vi "Get Slot Bus Device Function.vi"(0 "dwslot":u32, 5 "dwBus":u32, 7 "dwDevice":u32, 9 "dwFunction":u32, 11 "error in (no error)":errorcluster) -> (3 "function return":u32, 4 "dwslot out":u32, 6 "dwBus out":u32, 8 "dwDevice out":u32, 10 "dwFunction out":u32, 15 "error out":errorcluster)   [LabVIEW 2014, in "atmcd32d.lvlib"]
doc: "unsigned int WINAPI GetSlotBusDeviceFunction(DWORD * dwslot, DWORD * dwBus, DWORD * dwDevice, DWORD * dwFunction);"
uses:
  atmcd32d.lvlib
  atmcd32d.dll
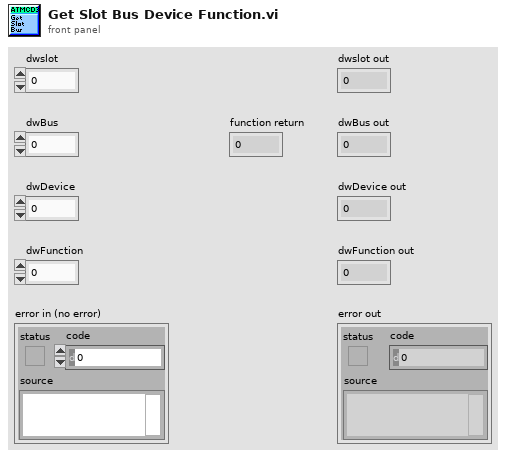
[diagram p1: front panel]
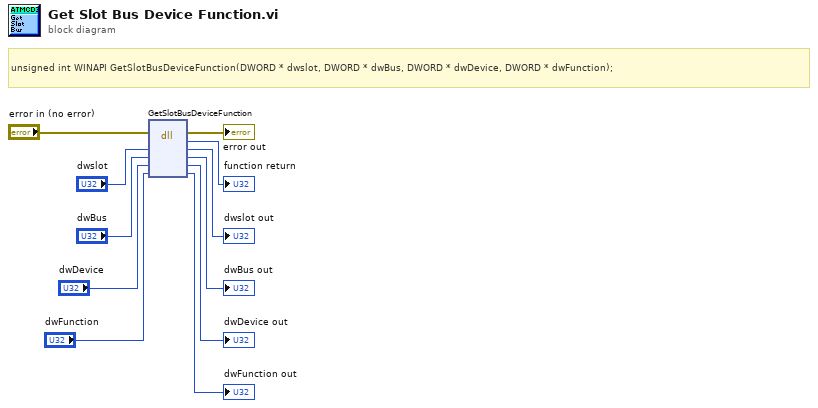
[diagram p0: block diagram]
diagram:
  # "unsigned int WINAPI GetSlotBusDeviceFunction(DWORD * dwslot, DWORD * dwBus, DWORD * dwDevice, DWORD * dwFunction);"
  n1 = dll-call lib="C:/Users/Bakir/Documents/Lambda2-Testing/lib/Andorlib/atmcd32d.*" fn="GetSlotBusDeviceFunction"(error in="error in (no error)", "dwslot"="dwslot", "dwBus"="dwBus", "dwDevice"="dwDevice", "dwFunction"="dwFunction") -> (error out=→"error out":errorcluster, →"function return":u32, "dwslot"=→"dwslot out":u32, "dwBus"=→"dwBus out":u32, "dwDevice"=→"dwDevice out":u32, "dwFunction"=→"dwFunction out":u32)  [unwired: 2 in, 1 out]
